vi "Init Moxa_2.vi"(9 "connect timeout ms":i32, 10 "port":u16, 11 "Address":string) -> (0 "error out":errorcluster, 2 "State":bool, 3 "Modbus Master out":refnum<class "Modbus Master.lvclass">)   [LabVIEW 2022 SP3]
doc: "Inits Moxa Device"
uses:
  <vilib>/NI/Modbus Library/API/Master/Modbus Master.lvclass
  <vilib>/NI/Modbus Library/API/Wrapper/Create TCP Master.vi
  <vilib>/NI/Modbus Library/API/Wrapper/API Main.lvlib
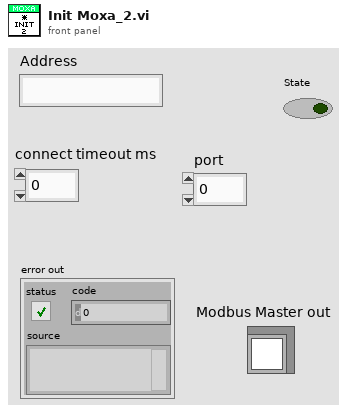
[diagram p1: front panel]
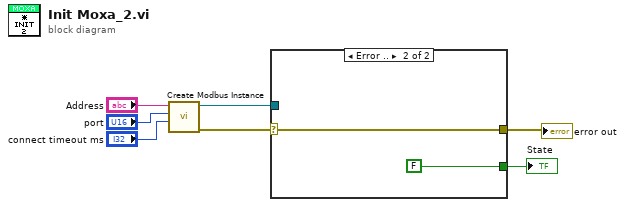
[diagram p0: block diagram]
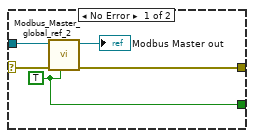
[diagram p2: hidden frame]
diagram:
  n1 = call-poly <vilib>:"Create Modbus Instance.vi"("connect timeout ms"="connect timeout ms", "port (502)"="port", "address"="Address") -> ("error out"=w3:errorcluster, "TCP master instance"=w4:refnum<class "Modbus Master.lvclass">)  [unwired: 7 in]
  n2 = case shown="Error .." w3 {
    selector: w3 -> [w10 w13]
    tunnel: w4 -> [w12 _]
    tunnel: [w9 FALSE ("State")] -> w2
    tunnel: [w8 w13] -> w1
    frame No Error {
      w9 = TRUE ("Read:F/Wirte:T")
      n3 = call "Modbus_Master_global_ref_2.vi"("Read:F/Wirte:T"=w9, "error in (no error) 2"=w10, "Modbus Master In"=w12) -> ("error out 2"=w8:errorcluster, "Modbus Master out"=→"Modbus Master out":refnum<class "Modbus Master.lvclass">)  [unwired: 7 in]
    }
    frame Error {
    }
  }
  "State" <- w2
  "error out" <- w1
